vi "test_Create MetaData Channel_single channel enumerated list.vi"(8 "error in (no error)":errorcluster, 11 "TestCase in":refnum<class "Instrument Addon Scripting API Channels Unit Tests.lvclass">) -> (0 "error out":errorcluster, 3 "TestCase out":refnum<class "Instrument Addon Scripting API Channels Unit Tests.lvclass">)   [LabVIEW 2019, in "Instrument Addon Scripting API Channels Unit Tests.lvclass"]
uses:
  Instrument Addon Scripting API Channels Unit Tests.lvclass
  <vilib>/addons/_JKI Toolkits/VI Tester/TestCase.llb/TestCase.lvclass
  APIs/Scripting API/TypeDefs/Single Channel Enumerated List Settings.ctl
  APIs/Scripting API/Instrument Addon Scripting API.lvlib
  <vilib>/NI VeriStand/Custom Device Tools/Custom Device Utility Library/Custom Device Utility Library.lvlib
  Addon/Addon Shared/SubVIs/Constants.vi
  Addon/Addon Shared/Instrument Addon Shared.lvlib
  Addon/Addon Shared/Types/FG Control.ctl
  <vilib>/NI VeriStand/Custom Device API/Custom Device API.lvlib
  <vilib>/NI VeriStand/Custom Device Tools/Custom Device Utility Library/NI VeriStand - Search for Item by Name.vi
  APIs/Scripting API/Channels/Create MetaData Channel - Single Channel - Enumerated List.vi
  <vilib>/NI VeriStand/Custom Device Tools/Custom Device Utility Library/NI VeriStand - Search for Item by GUID.vi
  C:/Program Files (x86)/National Instruments/LabVIEW 2019/vi.lib/addons/_JKI Toolkits/VI Tester/TestCase.llb/TestCase.lvclass
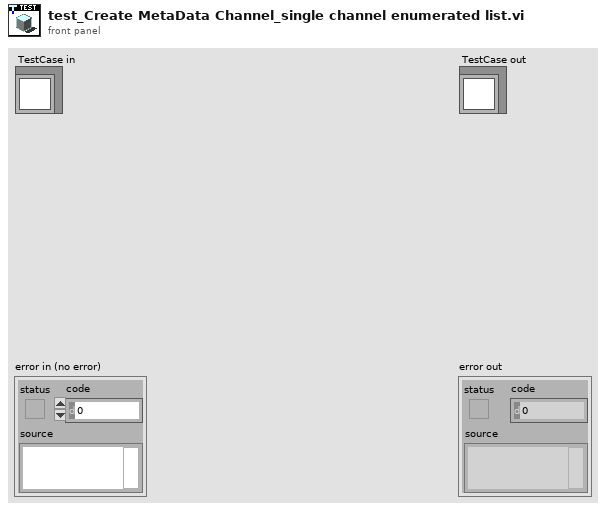
[diagram p1: front panel]
types:
  T1 = typedef "Instrument Addon Shared.lvlib/FG Control.ctl" = enum16{"Get", "Set"}
  T2 = typedef "Instrument Addon Scripting API.lvlib/Single Channel Enumerated List Settings.ctl" = cluster{"Enumerated List":string[], "Default Value":dbl, "Units":string}
  T3 = typedef "Custom Device API.lvlib/Custom Device Item Ref.ctl" = u64
  T4 = typedef "Instrument Addon Shared.lvlib/MetaData Parameters.ctl" = cluster{"Data Type":T5, "Channel Type":T6, "List":string[], "Format String":string, "Type":T7, "Delimiter":string, "Endian":T8}
  T5 = typedef "Instrument Addon Shared.lvlib/Protocol Data Type.ctl" = enum16{"Single Channel", "Array"}
  T6 = typedef "Instrument Addon Shared.lvlib/Metadata Channel Type.ctl" = enum16{"Enumerated List", "Format", "Type Cast"}
  T7 = typedef "Instrument Addon Shared.lvlib/Type Cast Type.ctl" = enum16{"DBL", "SGL", "U64", "U32", "U16", "U8", "I64", "I32", "I16", "I8"}
  T8 = typedef "Instrument Addon Shared.lvlib/Endian.ctl" = enum16{"Native", "Little", "Big"}
  T9 = typedef "Custom Device API.lvlib/Custom Device Channel.ctl" = cluster{"Type":T10, "Units":string, "Default Value":dbl, "Faultable":bool, "Scalable":bool}
  T10 = typedef "Custom Device API.lvlib/Custom Device Channel Type.ctl" = enum16{"Input", "Output"}
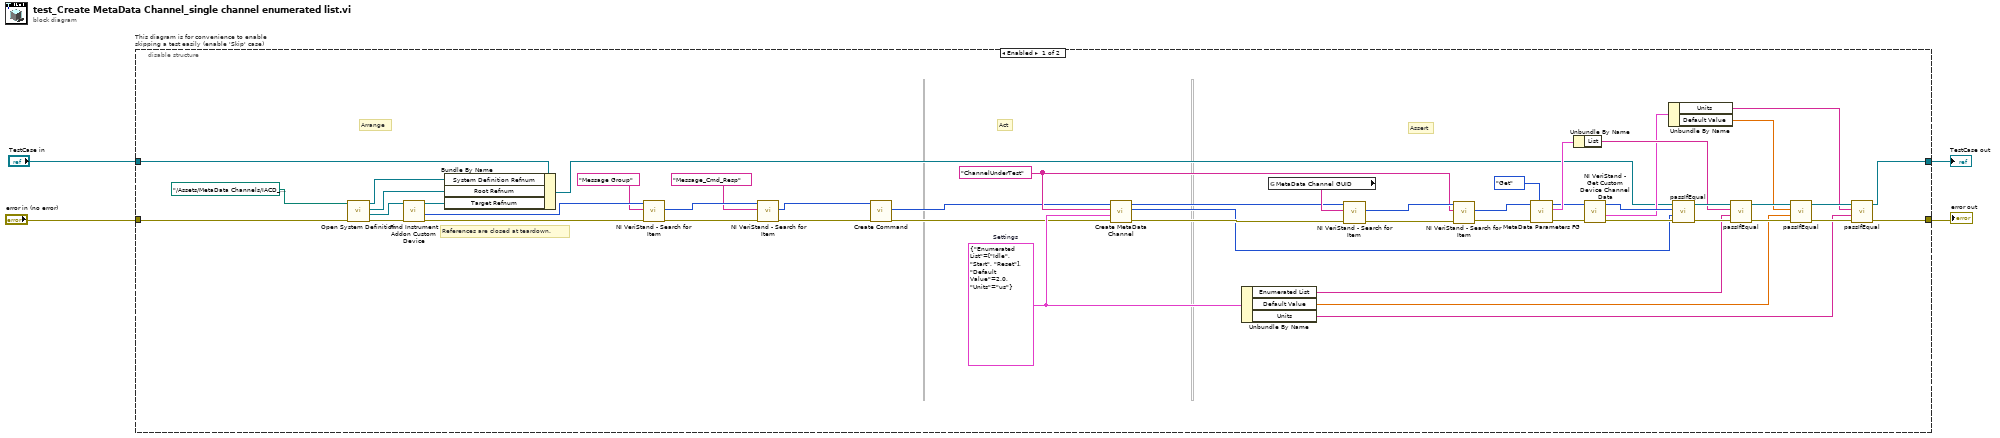
[diagram p0: block diagram]
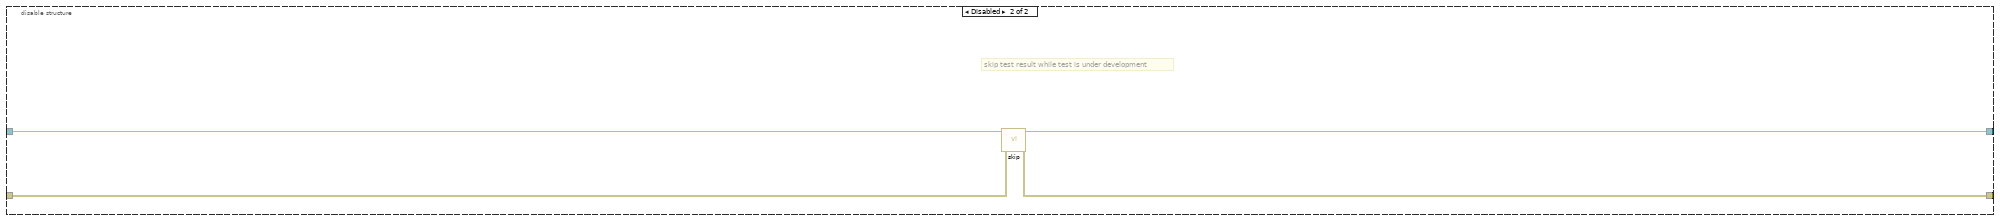
[diagram p2: hidden frame]
diagram:
  n1 = disable-structure "This diagram is for convenience to enable skipping a test easily (enable 'Skip' case)" shown="Enabled" {
    disable-tunnel: "TestCase in" -> [w21 w58]
    disable-tunnel: [w28 w56] -> w1
    disable-tunnel: [w27 w57] -> w3
    disable-tunnel: "error in (no error)" -> [w54 w55]
    frame Enabled {
      w20 = "ChannelUnderTest" ("Name")
      w19 = T2 {"Enumerated List"=["Idle", "Start", "Reset"], "Default Value"=2.0, "Units"="us"}  # Settings
      # "References are closed at teardown."
      # "Assert"
      # "Act"
      # "Arrange"
      n2 = call "Open System Definition.vi"("error in (no error)"=w54, "System Definition File"=path "../Assets/MetaData Channels/IACD_channels.nivssdf") -> ("error out"=w52:errorcluster, "Target Refnum"=w53:refnum<k24>, "Root Refnum"=w24:refnum<k24>, "System Definition Refnum"=w23:refnum<k24>)  [unwired: 6 in]
      n3 = call "Find Instrument Addon Custom Device.vi"("error in"=w52, "target in"=w53) -> ("error out"=w15:errorcluster, "NodeID"=w14:u64, "target out"=w25:refnum<k24>)  [unwired: 7 in]
      n4 = Bundle By Name(cluster=w21, "System Definition Refnum"=w23, "Root Refnum"=w24, "Target Refnum"=w25) -> (w22:refnum<class "Instrument Addon Scripting API Channels Unit Tests.lvclass">)
      n5 = call-poly <vilib>:"NI VeriStand - Search for Item.vi"("error in"=w15, "Item Name"="Message Group", "Section Ref in"=w14) -> ("error out"=w10:errorcluster, "Item Ref"=w12:T3)  [unwired: 5 in, 2 out]
      n6 = call-poly <vilib>:"NI VeriStand - Search for Item.vi"("error in"=w10, "Item Name"="Message_Cmd_Resp", "Section Ref in"=w12) -> ("error out"=w8:errorcluster, "Item Ref"=w6:T3)  [unwired: 5 in, 2 out]
      n7 = call "Create Command.vi"("error in"=w8, "message refnum In"=w6) -> ("error out"=w7:errorcluster, "command refnum"=w5:T3)  [unwired: 7 in, 1 out]
      n8 = call-poly "Create MetaData Channel.vi"("error in (no error)"=w7, "settings"=w19, "channel name"=w20, "command refnum in"=w5) -> ("error out"=w17:errorcluster, "channel refnum"=w16:T3, "command refnum out"=w18:T3)  [unwired: 5 in]
      n9 = Unbundle By Name(w19) -> ("Enumerated List"=w37:string[], "Default Value"=w33:dbl, "Units"=w32:string)
      n10 = global read "Constants.vi" "MetaData Channel GUID"() -> (w51:string)
      n11 = call-poly <vilib>:"NI VeriStand - Search for Item.vi"("error in"=w17, "Item GUID"=w51, "Section Ref in"=w18) -> ("error out"=w49:errorcluster, "Item Ref"=w50:T3)  [unwired: 5 in, 2 out]
      n12 = call-poly <vilib>:"NI VeriStand - Search for Item.vi"("error in"=w49, "Item Name"=w20, "Section Ref in"=w50) -> ("error out"=w48:errorcluster, "Item Ref"=w47:T3)  [unwired: 5 in, 2 out]
      n13 = call "MetaData Parameters FG.vi"("Action"=FG_Control."Get", "error in (no error)"=w48, "Item Ref in"=w47) -> ("error out"=w35:errorcluster, "MetaData Parameters"=w45:T4, "Item Ref out"=w36:T3)  [unwired: 6 in]
      n14 = Unbundle By Name(w45) -> ("List"=w38:string[])
      n15 = call <vilib>:"NI VeriStand - Get Custom Device Channel Data.vi"("error in (no error)"=w35, "Channel Ref in"=w36) -> ("error out"=w26:errorcluster, "Channel"=w31:T9, "Channel Ref out"=w34:T3)  [unwired: 4 in, 3 out]
      n16 = Unbundle By Name(w31) -> ("Units"=w29:string, "Default Value"=w30:dbl)
      n17 = call-dynamic "passIfEqual.vi"("error in (no error)"=w26, "y"=w16, "x"=w34, "TestCase in"=w22) -> ("error out"=w44:errorcluster, "TestCase out"=w43:refnum<class "Instrument Addon Scripting API Channels Unit Tests.lvclass">)  [unwired: 6 in]
      n18 = call-dynamic "passIfEqual.vi"("error in (no error)"=w44, "y"=w37, "x"=w38, "TestCase in"=w43) -> ("error out"=w42:errorcluster, "TestCase out"=w41:refnum<class "Instrument Addon Scripting API Channels Unit Tests.lvclass">)  [unwired: 6 in]
      n19 = call-dynamic "passIfEqual.vi"("error in (no error)"=w42, "y"=w33, "x"=w30, "TestCase in"=w41) -> ("error out"=w40:errorcluster, "TestCase out"=w39:refnum<class "Instrument Addon Scripting API Channels Unit Tests.lvclass">)  [unwired: 6 in]
      n20 = call-dynamic "passIfEqual.vi"("error in (no error)"=w40, "y"=w32, "x"=w29, "TestCase in"=w39) -> ("error out"=w27:errorcluster, "TestCase out"=w28:refnum<class "Instrument Addon Scripting API Channels Unit Tests.lvclass">)  [unwired: 6 in]
    }
    frame Disabled {
      # "skip test result while test is under development"
      n21 = call <vilib>:"skip.vi"("error in (no error)"=w55, "TestCase in"=w58) -> ("error out"=w57:errorcluster, "TestCase out"=w56:refnum<class "Instrument Addon Scripting API Channels Unit Tests.lvclass">)  [unwired: 8 in]
    }
  }
  "error out" <- w3
  "TestCase out" <- w1
